vi "Get Child Tag.vi"(10 "Sh Var Name in":string, 11 "VS Name in":string) -> (1 "Sh Var Name out":string, 2 "VS Name out":string, 3 "Child Tag":string)   [LabVIEW 2015, in "Shared Variable Custom Device.lvlib"]
uses:
  Shared Variable Custom Device.lvlib
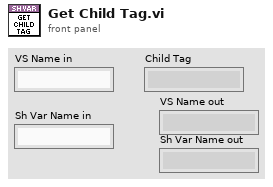
[diagram p1: front panel]
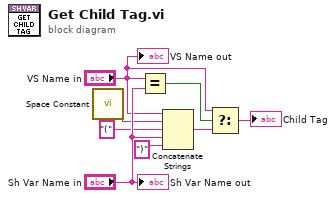
[diagram p0: block diagram]
diagram:
  n1 = call <vilib>:"Space Constant.vi"() -> ("String"=w3:string)
  n2 = Equal?(x="VS Name in", y="Sh Var Name in") -> (x = y?=w1:bool)
  n3 = Concatenate Strings("VS Name in", w3, "(" ("string"), "Sh Var Name in", ")" ("string")) -> (w7:string)
  n4 = Select(t="VS Name in", s=w1, f=w7) -> (s? t:f=→"Child Tag":string)
  "VS Name out" <- "VS Name in"
  "Sh Var Name out" <- "Sh Var Name in"
